vi "chart series set marker type.vi"(8 "error in (no error)":errorcluster, 10 "type":u8, 11 "series":u32) -> (0 "error out":errorcluster)   [LabVIEW 8.6]
doc: "void chart_series_set_marker_type(lxw_chart_series series, uint8_t type);"
uses:
  pending_lvxlsxwriter/xlsxwriter.dll
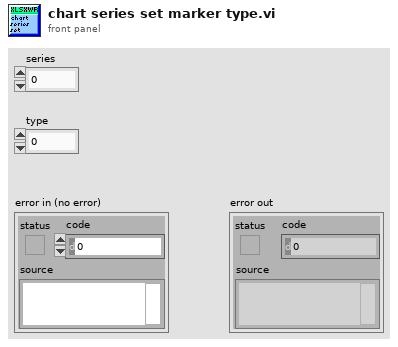
[diagram p1: front panel]
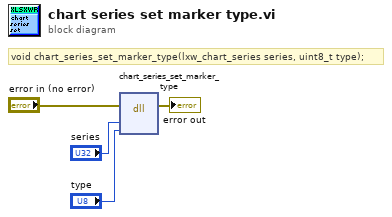
[diagram p0: block diagram]
diagram:
  # "void chart_series_set_marker_type(lxw_chart_series series, uint8_t type);"
  n1 = dll-call lib="C:/Users/WDAGUtilityAccount/Desktop/pending_lvxlsxwriter/xlsxwriter.*" fn="chart_series_set_marker_type"(error in="error in (no error)", "series"="series", "type"="type") -> (error out=→"error out":errorcluster)  [unwired: 5 in, 1 out]
